vi "I2C Message Buffer - Destroy.vi"(8 "error in (no error)":errorcluster) -> (0 "error out":errorcluster)   [LabVIEW 2025, in "I2C Bus Monitor.lvclass"]
uses:
  I2C Bus Monitor.lvclass
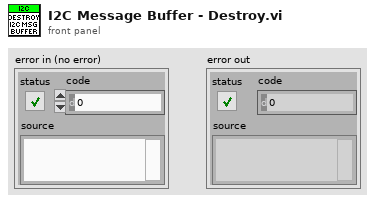
[diagram p1: front panel]
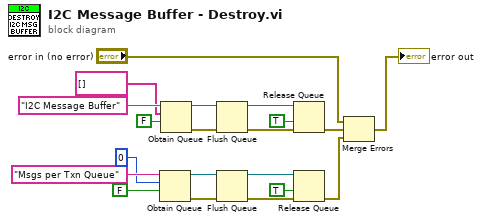
[diagram p0: block diagram]
diagram:
  n1 = Obtain Queue(name (unnamed)="Msgs per Txn Queue", element data type=0 ("max queue size (-1, unlimited)"), create if not found? (T)=FALSE) -> (queue out=w5:refnum<queue>, error out=w4:errorcluster)  [unwired: 2 in, 1 out]
  n2 = Obtain Queue(name (unnamed)="I2C Message Buffer", element data type=string[] [] ("I2C Messages"), create if not found? (T)=FALSE) -> (queue out=w13:refnum<queue>, error out=w19:errorcluster)  [unwired: 2 in, 1 out]
  n3 = Flush Queue(queue=w13, error in (no error)=w19) -> (queue out=w12:refnum<queue>, error out=w14:errorcluster)  [unwired: 1 out]
  n4 = Flush Queue(queue=w5, error in (no error)=w4) -> (queue out=w8:refnum<queue>, error out=w7:errorcluster)  [unwired: 1 out]
  n5 = Release Queue(queue=w12, force destroy? (F)=TRUE, error in (no error)=w14) -> (error out=w20:errorcluster)  [unwired: 2 out]
  n6 = Release Queue(queue=w8, force destroy? (F)=TRUE, error in (no error)=w7) -> (error out=w2:errorcluster)  [unwired: 2 out]
  n7 = Merge Errors("error in (no error)", w20, w2) -> (→"error out":errorcluster)
